vi "Error cluster to error response.vi"(8 "error in (no error)":errorcluster, 11 "response":string) -> (1 "err cluster":T1, 2 "JSON String":string, 3 "message":string)   [LabVIEW 2019, in "CommandResponse communication.lvlib"]
doc: "Converts standard LV error cluster to error response JSON string"
uses:
  CommandResponse communication.lvlib
  Error response.ctl
  <vilib>/Utility/error.llb/DialogType.ctl
  <userlib>/_OpenG.lib/string/string.llb/Trim Whitespace (String)__ogtk.vi
  <vilib>/addons/_JKI.lib/Serialization/JSON/JKI JSON Serialization.lvlib
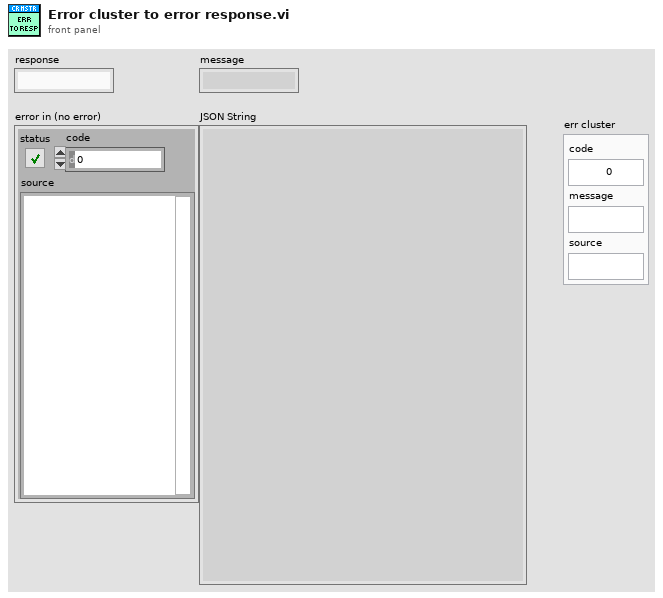
[diagram p1: front panel]
types:
  T1 = typedef "CommandResponse communication.lvlib/Error response.ctl" = cluster{"code":i32, "message":string, "source":string}
  T2 = typedef "DialogType.ctl" = u16
  T3 = typedef "TagReturnType.ctl" = enum16{"No Tag", "<err>", "<append>"}
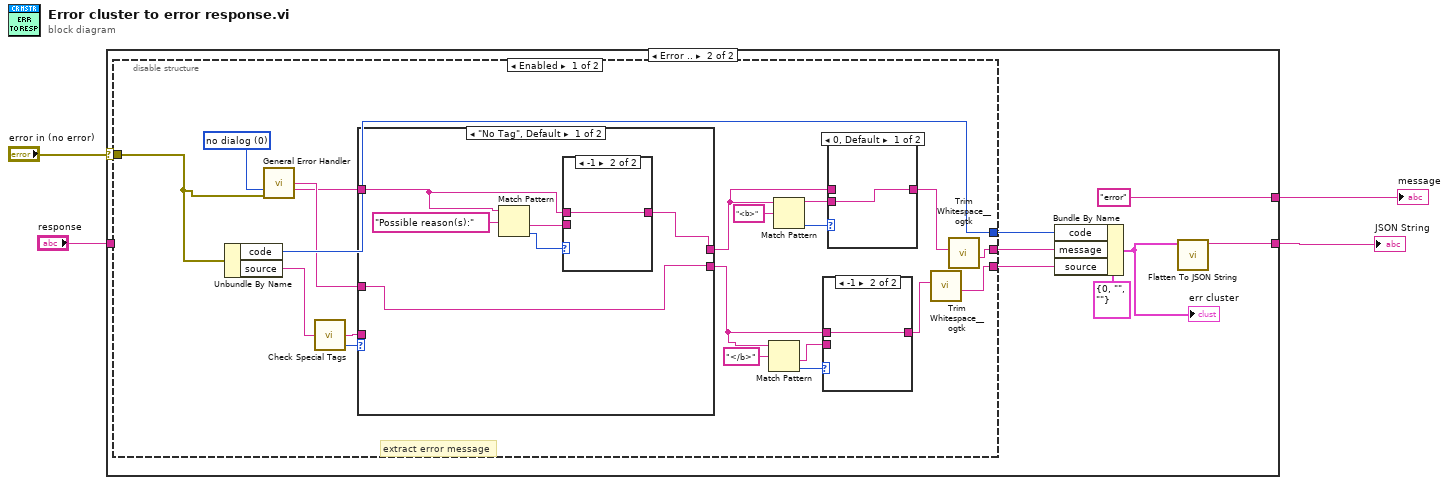
[diagram p0: block diagram]
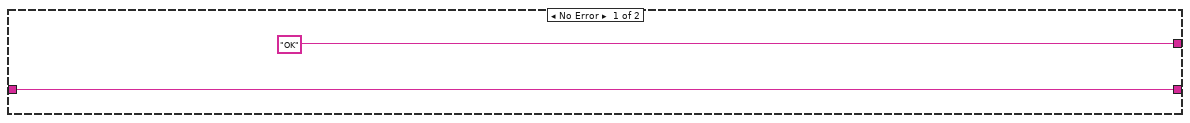
[diagram p2: hidden frame]
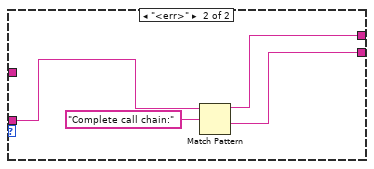
[diagram p6: hidden frame]
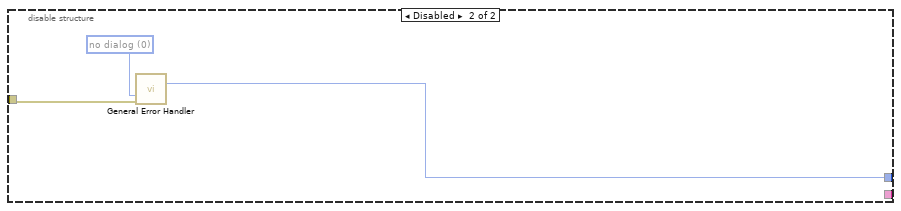
[diagram p7: hidden frame]
diagram:
  n1 = case shown="Error .." "error in (no error)" {
    selector: "error in (no error)" -> [_ w13]
    tunnel: ["OK" ("message") "error" ("message")] -> w1
    tunnel: [w5 w9] -> w3
    tunnel: "response" -> [w5 _]
    frame No Error {
    }
    frame Error {
      n2 = disable-structure shown="Enabled" {
        disable-tunnel: w13 -> [w32 w51]
        disable-tunnel: [w34 w53] -> w11
        disable-tunnel: [w22 _] -> w8
        disable-tunnel: [w17 _] -> w7
        frame Enabled {
          w33 = T2 0 items=["no dialog", "OK message", "continue or stop message", "OK message + warnings", "continue/stop + warnings"] ("type of dialog (OK msg:1)")
          # "extract error message"
          n3 = Unbundle By Name(w32) -> ("code"=w34:i32, "source"=w30:string)
          n4 = call <vilib>:"General Error Handler.vi"("type of dialog (OK msg:1)"=w33, "error in (no error)"=w32) -> ("source out"=w31:string, "message"=w15:string)  [unwired: 9 in, 3 out]
          n5 = call <vilib>:"Check Special Tags.vi"("source"=w30) -> ("After Tag (special data)"=w28:string, "Tag Found?"=w29:T3)  [unwired: 1 out]
          n6 = case shown="\"No Tag\", Default" w29 {
            tunnel: [w40 w48] -> w24
            tunnel: [w43 w47] -> w19
            tunnel: w31 -> [w43 _]
            tunnel: w28 -> [_ w49]
            tunnel: w15 -> [w39 _]
            frame "No Tag", Default {
              n7 = Match Pattern(string=w39, regular expression="Possible reason(s):") -> (after substring=w41:string, offset past match=w42:i32)  [unwired: 1 in, 2 out]
              n8 = case shown="-1" w42 {
                tunnel: [w45 w46] -> w40
                tunnel: w39 -> [_ w46]
                tunnel: w41 -> [w45 _]
                frame 0, Default {
                }
                frame -1 {
                }
              }
            }
            frame "<err>" {
              n9 = Match Pattern(string=w49, regular expression="Complete call chain:") -> (before substring=w48:string, after substring=w47:string)  [unwired: 1 in, 2 out]
            }
          }
          n10 = Match Pattern(string=w19, regular expression="</b>") -> (after substring=w16:string, offset past match=w21:i32)  [unwired: 1 in, 2 out]
          n11 = Match Pattern(string=w24, regular expression="<b>") -> (before substring=w23:string, offset past match=w26:i32)  [unwired: 1 in, 2 out]
          n12 = case shown="-1" w21 {
            tunnel: [w35 w36] -> w18
            tunnel: w19 -> [_ w36]
            tunnel: w16 -> [w35 _]
            frame 0, Default {
            }
            frame -1 {
            }
          }
          n13 = case shown="0, Default" w26 {
            tunnel: [w37 w38] -> w25
            tunnel: w24 -> [_ w38]
            tunnel: w23 -> [w37 _]
            frame 0, Default {
            }
            frame -1 {
            }
          }
          n14 = call-poly <userlib>:"Trim Whitespace__ogtk.vi"("String in"=w18) -> ("String out"=w17:string)  [unwired: 6 in]
          n15 = call-poly <userlib>:"Trim Whitespace__ogtk.vi"("String in"=w25) -> ("String out"=w22:string)  [unwired: 6 in]
        }
        frame Disabled {
          w52 = T2 0 items=["no dialog", "OK message", "continue or stop message", "OK message + warnings", "continue/stop + warnings"] ("type of dialog (OK msg:1)")
          n16 = call <vilib>:"General Error Handler.vi"("type of dialog (OK msg:1)"=w52, "error in (no error)"=w51) -> ("code out"=w53:i32)  [unwired: 9 in, 4 out]
        }
      }
      n17 = Bundle By Name(cluster=T1 {"code"=0, "message"="", "source"=""} ("Error response"), "code"=w11, "message"=w8, "source"=w7) -> (w10:T1)
      "err cluster" <- w10
      n18 = call <vilib>:"Flatten To JSON String.vi"("Variant"=w10) -> ("JSON String"=w9:string)  [unwired: 9 in, 1 out]
    }
  }
  "JSON String" <- w3
  "message" <- w1
